vi "KE_Acquire.vi"(2 "error in":T1, 3 "Type":u16(ring) items=["First", "Second"], 4 "INSTR_PARAM 2":refnum<vi>) -> (0 "error out":T1, 1 "Voltage":dbl)   [LabVIEW 2012]
uses:
  Controls/Instr_Param.ctl
  Controls/USB4000_Data.ctl
  KE236.LLB/Keith 236 Operate/Standby.vi
panel:
  in  "integration time (medium:1)":u16(ring)=1 items=["fast perod", "medium period", "line cycle period @ 50Hz", "line cycle period @ 60Hz"]
  out "?":T2(array[cluster])
  out "device dependent errors":string
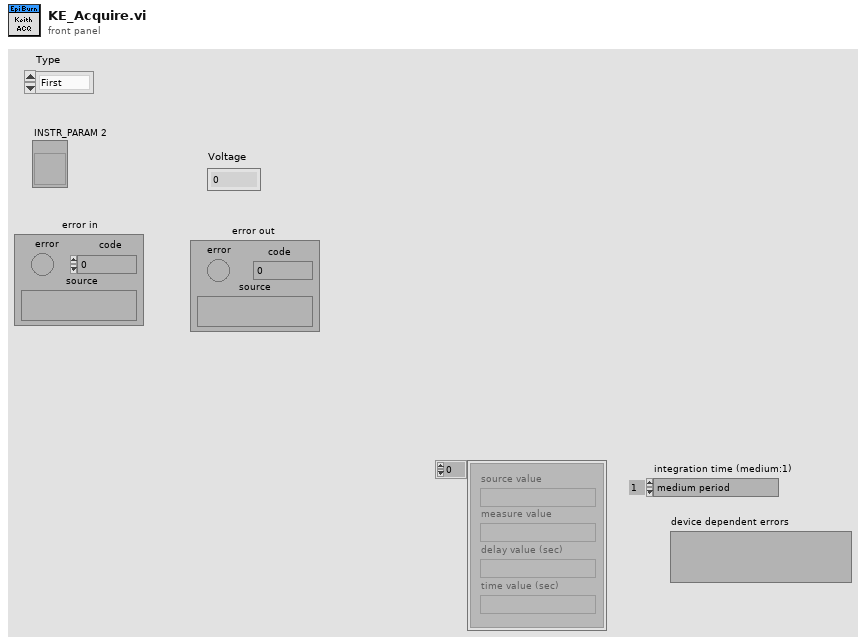
[diagram p1: front panel]
types:
  T1 = cluster{"error":bool, "code":i32, "source":string}
  T2 = cluster{"source value":string, "measure value":string, "delay value (sec)":string, "time value (sec)":string}[]
  T3 = typedef "Instr_Param.ctl" = cluster{"Keithley_Param":cluster{"Start Current,mA":dbl, "Stop Current,mA":dbl, "Voltage Compliance,V":dbl, "GPIB":string}, "USB4000_Param":cluster{"Integration Time":i32, "Wl min,nm":dbl, "Wl max,nm":dbl, "USB4000":T4}, "Ophir_Param":cluster{"VISA resource name":refnum<visa-resource-name>, "Calibration Wl":dbl}}
  T4 = typedef "USB4000_Data.ctl" = cluster{"Wrapper Out":u32, "Number of Spectrometers":i32, "Wavelength":dbl[], "EL Spectrum":dbl[], "Int Time (usec)":i32, bool, "Background":dbl[]}
  T5 = cluster{"Start Current,mA":dbl, "Stop Current,mA":dbl, "Voltage Compliance,V":dbl, "GPIB":string}
  T6 = cluster{"source value":string, "measure value":string, "delay value (sec)":string, "time value (sec)":string}
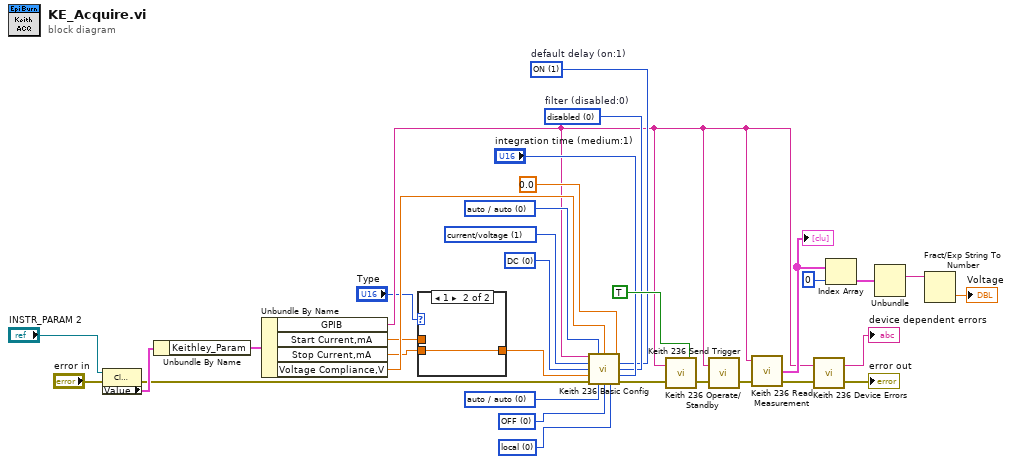
[diagram p0: block diagram]
diagram:
  w17 = u16 1 items=["OFF", "ON"]  # default delay (on:1)
  w18 = u16 0 items=["disabled", "2 readings", "4 readings", "8 readings", "16 readings", "32 readings"]  # filter (disabled:0)
  w21 = u16 0 items=["local", "remote"] ("sense (local:0)")
  w22 = u16 0 items=["OFF", "ON"] ("suppression (off:0)")
  w23 = u16 0 items=["auto / auto", "1 nA / 1.1 V", "10 nA / 11 V", "100 nA / 110 V", "0.001 mA / 110 V", "0.01 mA / 110 V", "0.1 mA / 110 V", "1 mA / 110 V", "10 mA / 110 V", "100 mA / 110 V"] ("compliance/\nmeasurement range (auto:0)")
  w24 = u16 0 items=["DC", "sweep"] ("function (DC:0)")
  w25 = u16 1 items=["voltage/current", "current/voltage"] ("source/measure (V/I:0)")
  w26 = u16 0 items=["auto / auto", "1 nA / 1.1 V", "10 nA / 11 V", "100 nA / 110 V", "0.001 mA / 110 V", "0.01 mA / 110 V", "0.1 mA / 110 V", "1 mA / 110 V", "10 mA / 110 V", "100 mA / 110 V"] ("source range\nI source / V source (auto:0)")
  n1 = property class="Clust (strict)"(reference="INSTR_PARAM 2", error in="error in") -> (error out=w1:errorcluster, "Value"=w3:T3)  [unwired: 1 out]
  n2 = Unbundle By Name(w3) -> ("Keithley_Param"=w27:T5)
  n3 = Unbundle By Name(w27) -> ("GPIB"=w9:string, "Start Current,mA"=w7:dbl, "Stop Current,mA"=w6:dbl, "Voltage Compliance,V"=w16:dbl)
  n4 = case shown="1" "Type" {
    tunnel: w7 -> [w34 _]
    tunnel: w6 -> [_ w35]
    tunnel: [w34 w35] -> w5
    frame 0, Default {
    }
    frame 1 {
    }
  }
  n5 = call "Keith 236 Basic Config.vi"("GPIB address"=w9, "source range\nI source / V source (auto:0)"=w26, "voltage \ncompliance level"=w16, "DC delay (sec)"=0.0, "source/measure (V/I:0)"=w25, "default delay (on:1)"=w17, "function (DC:0)"=w24, "filter (disabled:0)"=w18, "source level"=w5, "integration time (medium:1)"="integration time (medium:1)", "error in"=w1, "compliance/\nmeasurement range (auto:0)"=w23, "suppression (off:0)"=w22, "sense (local:0)"=w21) -> ("error out"=w15:T1)  [unwired: 1 in]
  n6 = call "Keith 236 Operate/Standby.vi"("source"=TRUE, "error in"=w15, "GPIB address"=w9) -> ("error out"=w30:T1)
  n7 = call "Keith 236 Send Trigger.vi"("GPIB address"=w9, "error in"=w30) -> ("error out"=w32:T1)
  n8 = call "Keith 236 Read Measurement.vi"("error in"=w32, "GPIB address"=w9) -> ("error out"=w33:T1, "display"=w14:T2)  [unwired: 2 out]
  "?" <- w14
  n9 = call "Keith 236 Device Errors.vi"("error in"=w33, "GPIB address"=w9) -> ("error out"=→"error out":T1, "device dependent errors"=→"device dependent errors":string)
  n10 = Index Array(array=w14, index=0) -> (element=w12:T6)
  n11 = Unbundle(w12) -> ("measure value"=w11:string)  [unwired: 3 out]
  n12 = Fract/Exp String To Number(string=w11) -> (number=→"Voltage":dbl)  [unwired: 3 in, 1 out]
